vi "TestExec.Configure Reports, Lookup Rpt Dir.vi"(10 "Seq Name":string, 11 "Seq_Dir":cluster{"Sequence":string, "Folder":path}[](array[cluster])) -> (2 "Valid":bool, 3 "Folder":path)   [LabVIEW 2019]
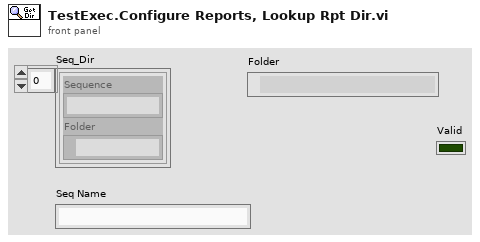
[diagram p1: front panel]
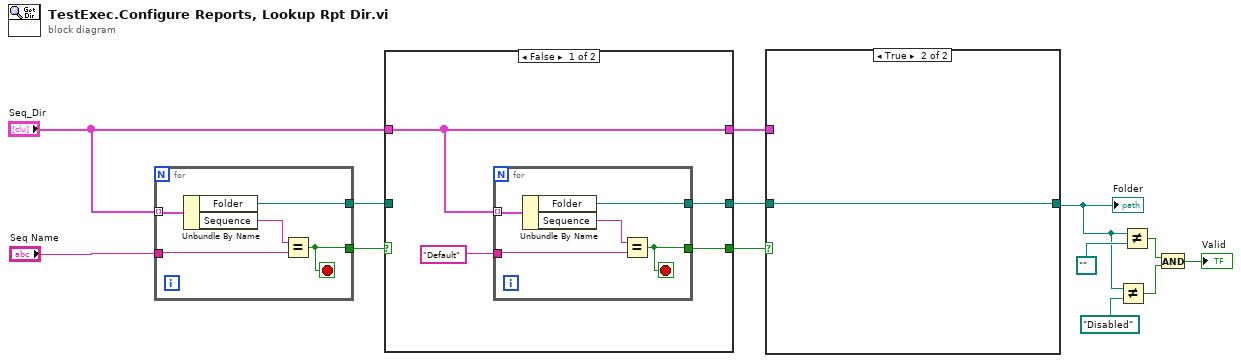
[diagram p0: block diagram]
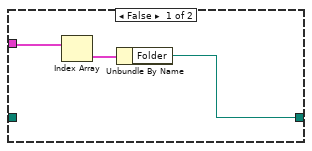
[diagram p2: hidden frame]
diagram:
  n1 = for {
    tunnel: "Seq_Dir" -> [w18] mode=indexing
    tunnel: "Seq Name" -> [w16]
    tunnel: [w15] -> w11
    tunnel: [w14] -> w10
    stop <- w15 stop-if-true
    n2 = Unbundle By Name(w18) -> ("Folder"=w14:path, "Sequence"=w17:string)
    n3 = Equal?(x=w17, y=w16) -> (x = y?=w15:bool)
  }
  n4 = case shown="False" w11 {
    selector: w11 -> [_ w29]
    tunnel: "Seq_Dir" -> [w19 w28]
    tunnel: w10 -> [_ w30]
    tunnel: [w21 w30] -> w8
    tunnel: [w20 w29] -> w9
    tunnel: [w19 w28] -> w7
    frame False {
      n5 = for {
        tunnel: w19 -> [w27] mode=indexing
        tunnel: "Default" -> [w25]
        tunnel: [w24] -> w20
        tunnel: [w23] -> w21
        stop <- w24 stop-if-true
        n6 = Unbundle By Name(w27) -> ("Folder"=w23:path, "Sequence"=w26:string)
        n7 = Equal?(x=w26, y=w25) -> (x = y?=w24:bool)
      }
    }
    frame True {
    }
  }
  n8 = case shown="True" w9 {
    tunnel: w8 -> [_ w34]
    tunnel: [w31 w34] -> w4
    tunnel: w7 -> [w33 _]
    frame False {
      n9 = Index Array(array=w33) -> (element=w32:cluster{"Sequence":string, "Folder":path})  [unwired: 1 in]
      n10 = Unbundle By Name(w32) -> ("Folder"=w31:path)
    }
    frame True {
    }
  }
  "Folder" <- w4
  n11 = Not Equal?(x=w4, y=path "Disabled") -> (x != y?=w2:bool)
  n12 = Not Equal?(x=w4, y=path "") -> (x != y?=w3:bool)
  n13 = And(x=w3, y=w2) -> (x .and. y?=→"Valid":bool)
